vi "iTCset.vi"(8 "error in (no error)":errorcluster, 9 "Set Point":dbl min=0.0 max=100.0 step=0.01, 10 "iTCSetCtrl":T1, 11 "VISA resource name":refnum<visa-resource-name>) -> (0 "error out":errorcluster, 1 "read buffer":string, 2 "number":dbl, 3 "VISA resource name out":refnum<visa-resource-name>)   [LabVIEW 2017]
uses:
  controls/iTCsetCtrl.ctl
  <vilib>/regexp/Match Regular Expression.xnode
panel:
  in  "Set":bool
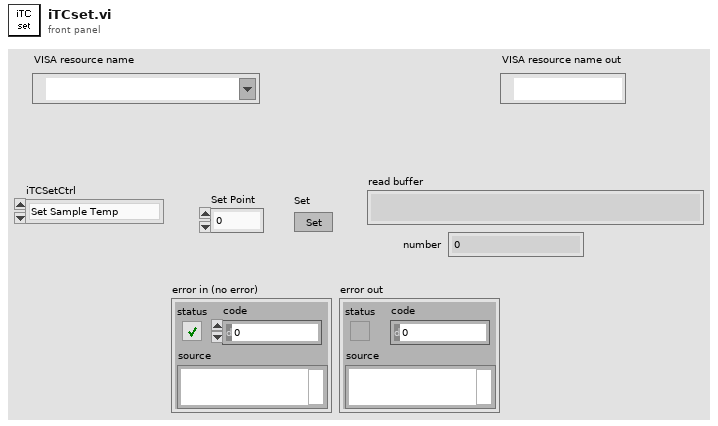
[diagram p1: front panel]
types:
  T1 = typedef "iTCsetCtrl.ctl" = enum16{"Set Sample Temp", "Set VTI Temp", "Set Needle Valve", "Set VTI Heater Power", "Set Sample Heater Power", "Set VTI Pressure"}
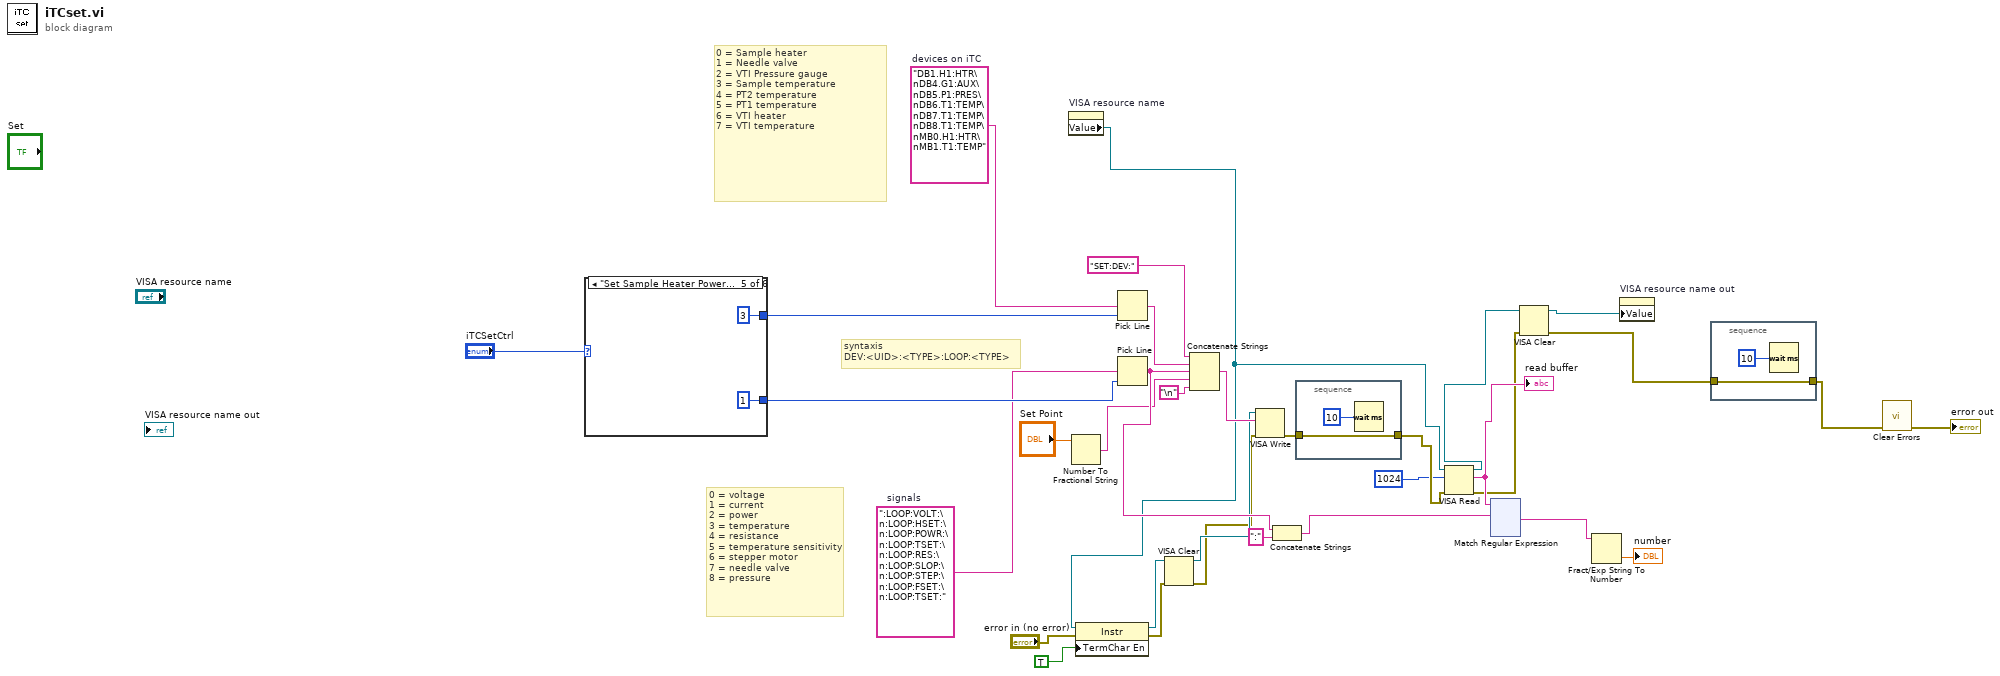
[diagram p0: block diagram]
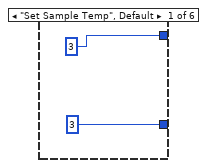
[diagram p2: hidden frame]
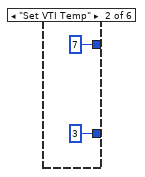
[diagram p3: hidden frame]
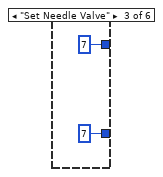
[diagram p4: hidden frame]
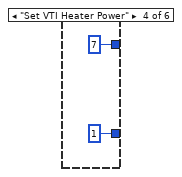
[diagram p5: hidden frame]
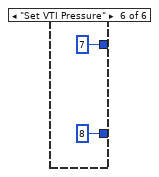
[diagram p6: hidden frame]
diagram:
  w19 = ":LOOP:VOLT:\n:LOOP:HSET:\n:LOOP:POWR:\n:LOOP:TSET:\n:LOOP:RES:\n:LOOP:SLOP:\n:LOOP:STEP:\n:LOOP:FSET:\n:LOOP:TSET:"  # signals
  w17 = "DB1.H1:HTR\nDB4.G1:AUX\nDB5.P1:PRES\nDB6.T1:TEMP\nDB7.T1:TEMP\nDB8.T1:TEMP\nMB0.H1:HTR\nMB1.T1:TEMP"  # devices on iTC
  # "0 = Sample heater\n1 = Needle valve\n2 = VTI Pressure gauge\n3 = Sample temperature\n4 = PT2 temperature\n5 = PT1 temperature\n6 = VTI heater\n7 = VTI temperature"
  # "0 = voltage\n1 = current\n2 = power\n3 = temperature\n4 = resistance\n5 = temperature sensitivity\n6 = stepper motor\n7 = needle valve\n8 = pressure"
  # "syntaxis\nDEV:<UID>:<TYPE>:LOOP:<TYPE>"
  n1 = case shown="\"Set Sample Heater Power\"" "iTCSetCtrl" {
    tunnel: [3 ("line index") 7 ("line index") 7 ("line index") 7 ("line index") 3 ("line index") 7 ("line index")] -> w27
    tunnel: [3 ("line index") 3 ("line index") 7 ("line index") 1 ("line index") 1 ("line index") 8 ("line index")] -> w28
    frame "Set Sample Temp", Default {
    }
    frame "Set VTI Temp" {
    }
    frame "Set Needle Valve" {
    }
    frame "Set VTI Heater Power" {
    }
    frame "Set Sample Heater Power" {
    }
    frame "Set VTI Pressure" {
    }
  }
  n2 = property on="VISA resource name" class="VISAName"() -> ("Value"=w9:refnum<visa-resource-name>)  [unwired: 2 in, 2 out]
  n3 = Number To Fractional String(number="Set Point") -> (F-format string=w14:string)  [unwired: 3 in]
  n4 = property class="Instr"(reference=w9, error in="error in (no error)", "TermChar En"=TRUE ("Message Based Settings:Termination Character Enable")) -> (reference out=w8:refnum<visa-resource-name>, error out=w7:errorcluster)
  n5 = Pick Line(multi-line string=w17, line index=w27) -> (output string=w23:string)  [unwired: 1 in]
  n6 = Pick Line(multi-line string=w19, line index=w28) -> (output string=w25:string)  [unwired: 1 in]
  n7 = VISA Clear(VISA resource name=w8, error in (no error)=w7) -> (VISA resource name out=w10:refnum<visa-resource-name>, error out=w6:errorcluster)
  n8 = Concatenate Strings("SET:DEV:" ("write buffer"), w23, w25, w14, "\n") -> (w24:string)
  n9 = VISA Write(VISA resource name=w10, write buffer=w24, error in (no error)=w6) -> (error out=w22:errorcluster)  [unwired: 2 out]
  n10 = Concatenate Strings(w25, ":" ("string")) -> (w26:string)
  n11 = stacked-sequence {
    tunnel: w22 -> [w47]
    tunnel: [w47] -> w31
    frame #0 {
      n12 = Wait (ms)(milliseconds to wait=u32 10) -> ()  [unwired: 1 out]
    }
  }
  n13 = VISA Read(VISA resource name=w9, byte count=u32 1024, error in (no error)=w31) -> (VISA resource name out=w5:refnum<visa-resource-name>, read buffer=w32:string, error out=w3:errorcluster)  [unwired: 1 out]
  "read buffer" <- w32
  n14 = xnode "Match Regular Expression"("input string"=w32, "regular expression"=w26) -> ("after match"=w29:string)  [unwired: 4 in, 4 out]
  n15 = VISA Clear(VISA resource name=w5, error in (no error)=w3) -> (VISA resource name out=w4:refnum<visa-resource-name>, error out=w2:errorcluster)
  n16 = Fract/Exp String To Number(string=w29) -> (number=→"number":dbl)  [unwired: 3 in, 1 out]
  n17 = property on="VISA resource name out" class="VISAName"("Value"=w4) -> ()  [unwired: 2 in, 2 out]
  n18 = stacked-sequence {
    tunnel: w2 -> [w48]
    tunnel: [w48] -> w1
    frame #0 {
      n19 = Wait (ms)(milliseconds to wait=u32 10) -> ()  [unwired: 1 out]
    }
  }
  n20 = call <vilib>:"Clear Errors.vi"("error in (no error)"=w1) -> ("error out"=→"error out":errorcluster)  [unwired: 5 in, 1 out]
